vi "Autonomous Independent.vi"() -> ()   [LabVIEW 2016]
doc: "This VI is called when autonomous begins, and will automatically be terminated when autonomous ends. You can carry out timed or sensor driven robot movement independently without needing to return to the caller."
uses:
  <vilib>/Rock Robotics/WPI/Utilities/WPI_GetSetVariantRefNum.vi
  <vilib>/Rock Robotics/Network Tables/NT Read String.vi
  Robot Global Data.vi
  <vilib>/addons/control/pid/pid.llb/PID (DBL).vi
  <vilib>/Rock Robotics/Network Tables/NT Write Numeric Array.vi
  <vilib>/addons/control/pid/NI_PID_pid.lvlib
panel:
  in  "Type":bool
  in  "Range V":cluster{"output high":dbl, "output low":dbl}={"output high"=100.0, "output low"=-100.0} {"output low" format="%.2f"; "output high" format="%.2f"}
  in  "PID gains V":T1={"proportional gain (Kc)"=1.0, "integral time (Ti, min)"=0.01, "derivative time (Td, min)"=0.0} {"derivative time (Td, min)" format="%.3f"; "integral time (Ti, min)" format="%.3f"; "proportional gain (Kc)" format="%.3f"}
  in  "Range P":cluster{"output high":dbl, "output low":dbl}={"output high"=100.0, "output low"=-100.0} {"output low" format="%.2f"; "output high" format="%.2f"}
  in  "PID gains P":T1={"proportional gain (Kc)"=1.0, "integral time (Ti, min)"=0.01, "derivative time (Td, min)"=0.0} {"derivative time (Td, min)" format="%.3f"; "integral time (Ti, min)" format="%.3f"; "proportional gain (Kc)" format="%.3f"}
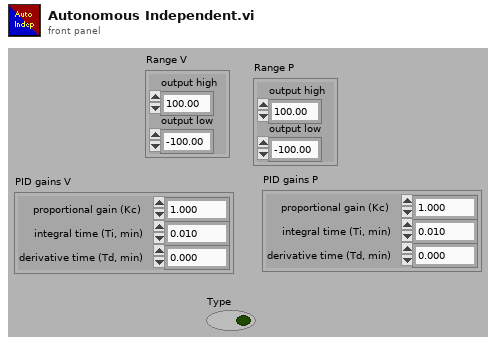
[diagram p1: front panel]
types:
  T1 = cluster{"proportional gain (Kc)":dbl, "integral time (Ti, min)":dbl, "derivative time (Td, min)":dbl}
  T2 = typedef "WPI_JoystickDevRef.ctl" = cluster{"Device":T3}
  T3 = typedef "WPI_JoystickDeviceEnum.ctl" = enum16{"USB 0", "USB 1", "USB 2", "USB 3", "USB 4", "USB 5"}
  T4 = typedef "WPI_EncoderDevRef.ctl" = cluster{"DevStatus":errorcluster, "EncoderIndex":T5, "CounterIndex":T6, "DistancePerCount":dbl, "Decoding Type":T7}
  T5 = typedef "FPGA_EncoderIdx.ctl" = enum8{"Enc 0", "Enc 1", "Enc 2", "Enc 3", "Enc 4", "Enc 5", "Enc 6", "Enc 7", "Invalid"}
  T6 = typedef "FPGA_CounterCtrSystemIndex.ctl" = enum8{"Ctr 0", "Ctr 1", "Ctr 2", "Ctr 3", "Ctr 4", "Ctr 5", "Ctr 6", "Ctr 7", "Invalid"}
  T7 = typedef "WPI_EncoderType.ctl" = enum16{"1x", "2x", "4x"}
  T8 = typedef "WPI_RobotDriveDevRef.ctl" = cluster{"DevStatus":errorcluster, "Motors[]":T9[], "Square Inputs":bool, "Max Output":dbl}
  T9 = typedef "WPI_MotorControlDeviceRef.ctl" = cluster{"DeviceStatus":errorcluster, "Type":T10, "PWM":cluster{"PWM Channel":T11, "DeadBand":T12}, "CAN":cluster{"Device Number":u8, "SetOutput VI Ref":variant, "GetOutput VI Ref":variant, "Enable VI Ref":variant, "Disable VI Ref":variant, "Data":variant}, "Invert":bool}
  T10 = typedef "WPI_MotorControlType.ctl" = enum16{"PWM", "CAN"}
  T11 = typedef "FPGA_DIOPWMChannel.ctl" = enum8{"PWM 0", "PWM 1", "PWM 2", "PWM 3", "PWM 4", "PWM 5", "PWM 6", "PWM 7", "PWM 8", "PWM 9", "PWM MXP 0", "PWM MXP 1", "PWM MXP 2", "PWM MXP 3", "PWM MXP 4", "PWM MXP 5", "PWM MXP 6", "PWM MXP 7", "PWM MXP 8", "PWM MXP 9", "Invalid"}
  T12 = typedef "WPI_PWMDeadband.ctl" = cluster{"Name":string, "maxPositivePwm":i32, "minPositivePwm":i32, "centerPwm":i32, "maxNegativePwm":i32, "minNegativePwm":i32, "angularRange":u16}
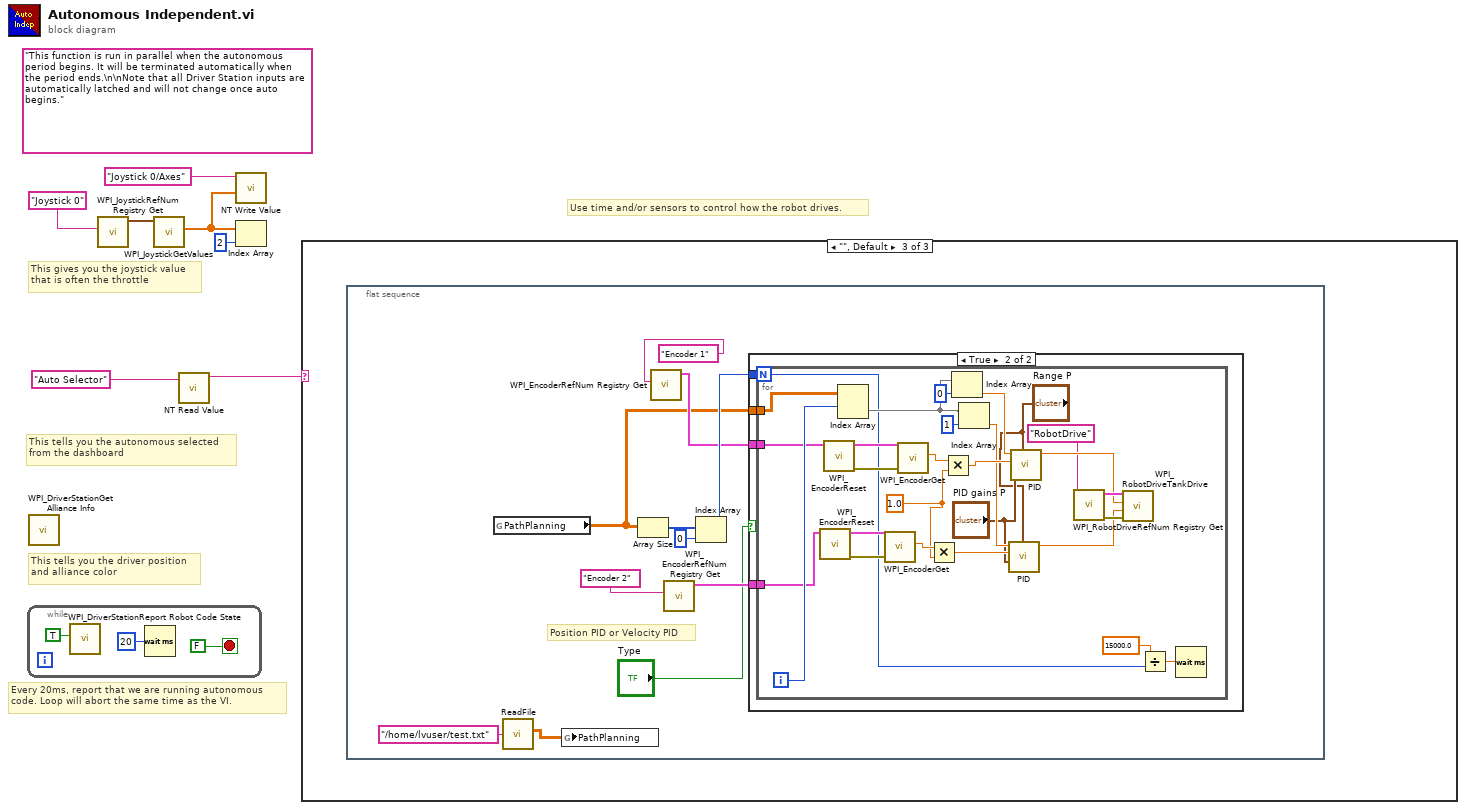
[diagram p0: block diagram]
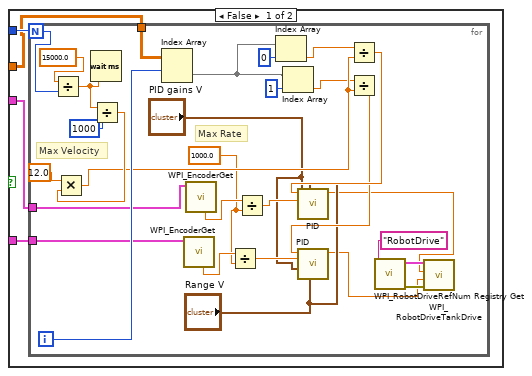
[diagram p4: hidden frame]
diagram:
  (unwired) "This function is run in parallel when the autonomous period begins. It will be terminated automatically when the period ends.\n\nNote that all Driver Station inputs are automatically latched and will not change once auto begins."
  # "This tells you the autonomous selected\nfrom the dashboard"
  # "Every 20ms, report that we are running autonomous\ncode. Loop will abort the same time as the VI."
  # "This gives you the joystick value\nthat is often the throttle"
  # "Use time and/or sensors to control how the robot drives."
  # "This tells you the driver position\nand alliance color"
  n1 = while {
    stop <- FALSE stop-if-true
    n2 = call <vilib>:"WPI_DriverStationReport Robot Code State.vi"("Autonomous"=TRUE) -> ()  [unwired: 10 in, 1 out]
    n3 = Wait (ms)(milliseconds to wait=u32 20) -> ()  [unwired: 1 out]
  }
  n4 = call <vilib>:"WPI_DriverStationGet Alliance Info.vi"() -> ()  [unwired: 12 out]
  n5 = call <vilib>:"WPI_JoystickRefNum Registry Get.vi"("refnum name"="Joystick 0") -> ("JoystickDevRef"=w6:T2)  [unwired: 1 in, 9 out]
  n6 = call <vilib>:"WPI_JoystickGetValues.vi"("JoystickDevRef"=w6) -> ("Axes"=w2:dbl[])  [unwired: 6 in, 4 out]
  n7 = call-poly <vilib>:"NT Read Value.vi"("Name"="Auto Selector") -> ("String"=w3:string)  [unwired: 9 in, 1 out]
  n8 = call-poly <vilib>:"NT Write Value.vi"("Numeric Array"=w2, "Name"="Joystick 0/Axes") -> ()  [unwired: 9 in, 1 out]
  n9 = Index Array(array=w2, index=2) -> ()  [unwired: 1 out]
  n10 = case shown="\"\", Default" w3 {
    frame "Alternative 1" {
    }
    frame "Alternative 2" {
    }
    frame "", Default {
      n11 = flat-sequence {
        frame #0 {
          # "Position PID or Velocity PID"
          n12 = global read "Robot Global Data.vi" "PathPlanning"() -> (w13:dbl[][])
          n13 = call "ReadFile.vi"("Location"="/home/lvuser/test.txt") -> ("Array - Numeric"=w11:dbl[][])  [unwired: 10 in]
          n14 = global write "Robot Global Data.vi" "PathPlanning"(w11) -> ()
          n15 = Array Size(array=w13) -> (size(s)=w21:i32[])
          n16 = call <vilib>:"WPI_EncoderRefNum Registry Get.vi"("refnum name"="Encoder 1") -> ("EncoderDevRef"=w17:T4)  [unwired: 9 in, 1 out]
          n17 = call <vilib>:"WPI_EncoderRefNum Registry Get.vi"("refnum name"="Encoder 2") -> ("EncoderDevRef"=w15:T4)  [unwired: 9 in, 1 out]
          n18 = Index Array(array=w21, index=0) -> (element=w19:i32)
          n19 = case shown="True" "Type" {
            tunnel: w13 -> [w24 w59]
            tunnel: w19 -> [w25 w58]
            tunnel: w17 -> [w23 w57]
            tunnel: w15 -> [w22 w56]
            frame False {
              n20 = for {
                N: w25 -> [w54]
                tunnel: w24 -> [w51]
                tunnel: w23 -> [w38]
                tunnel: w22 -> [w37]
                i -> [w50]
                w39 = 1000.0
                # "Max Rate"
                # "Max Velocity"
                n21 = Divide(x=15000.0, y=w54) -> (x/y=w48:dbl)
                n22 = Wait (ms)(milliseconds to wait=w48) -> ()  [unwired: 1 out]
                n23 = Divide(x=w48, y=1000) -> (x/y=w46:dbl)
                n24 = Multiply(x=12.0, y=w46) -> (x*y=w45:dbl)
                n25 = Index Array(array=w51, index (row)=w50) -> (element=w44:dbl[])  [unwired: 1 in]
                n26 = call <vilib>:"WPI_EncoderGet.vi"("EncoderDevRef"=w37) -> ("Rate"=w40:dbl)  [unwired: 5 in, 5 out]
                n27 = call <vilib>:"WPI_EncoderGet.vi"("EncoderDevRef"=w38) -> ("Rate"=w41:dbl)  [unwired: 5 in, 5 out]
                n28 = Divide(x=w40, y=w39) -> (x/y=w35:dbl)
                n29 = Divide(x=w41, y=w39) -> (x/y=w36:dbl)
                n30 = Index Array(array=w44, index=0) -> (element=w43:dbl)
                n31 = Index Array(array=w44, index=1) -> (element=w42:dbl)
                n32 = Divide(x=w43, y=w45) -> (x/y=w34:dbl)
                n33 = call-poly <vilib>:"PID.vi"("output range"="Range V", "PID gains"="PID gains V", "process variable"=w36, "setpoint"=w34) -> ("output"=w27:dbl)  [unwired: 6 in, 1 out]
                n34 = Divide(x=w42, y=w45) -> (x/y=w33:dbl)
                n35 = call-poly <vilib>:"PID.vi"("output range"="Range V", "PID gains"="PID gains V", "process variable"=w35, "setpoint"=w33) -> ("output"=w26:dbl)  [unwired: 6 in, 1 out]
                n36 = call <vilib>:"WPI_RobotDriveRefNum Registry Get.vi"("refnum name"="RobotDrive") -> ("error out"=w30:errorcluster, "RobotDriveDevRef"=w29:T8)  [unwired: 9 in]
                n37 = call <vilib>:"WPI_RobotDriveTankDrive.vi"("error in (no error)"=w30, "Right axis value"=w26, "Left axis value"=w27, "RobotDriveDevRef"=w29) -> ()  [unwired: 5 in, 3 out]
              }
            }
            frame True {
              n38 = for {
                N: w58 -> [w63]
                tunnel: w59 -> [w78]
                tunnel: w57 -> [w61]
                tunnel: w56 -> [w60]
                i -> [w77]
                w85 = 1.0
                n39 = call <vilib>:"WPI_EncoderReset.vi"("EncoderDevRef"=w60) -> ("error out"=w83:errorcluster, "EncoderDevRef"=w84:T4)  [unwired: 9 in]
                n40 = call <vilib>:"WPI_EncoderReset.vi"("EncoderDevRef"=w61) -> ("error out"=w81:errorcluster, "EncoderDevRef"=w82:T4)  [unwired: 9 in]
                n41 = Index Array(array=w78, index (row)=w77) -> (element=w74:dbl[])  [unwired: 1 in]
                n42 = call <vilib>:"WPI_EncoderGet.vi"("error in (no error)"=w83, "EncoderDevRef"=w84) -> ("Distance"=w86:dbl)  [unwired: 4 in, 5 out]
                n43 = call <vilib>:"WPI_EncoderGet.vi"("error in (no error)"=w81, "EncoderDevRef"=w82) -> ("Distance"=w87:dbl)  [unwired: 4 in, 5 out]
                n44 = Multiply(x=w86, y=w85) -> (x*y=w80:dbl)
                n45 = Multiply(x=w87, y=w85) -> (x*y=w79:dbl)
                n46 = Index Array(array=w74, index=0) -> (element=w73:dbl)
                n47 = Index Array(array=w74, index=1) -> (element=w72:dbl)
                n48 = call-poly <vilib>:"PID.vi"("output range"="Range P", "PID gains"="PID gains P", "process variable"=w80, "setpoint"=w72) -> ("output"=w67:dbl)  [unwired: 6 in, 1 out]
                n49 = call-poly <vilib>:"PID.vi"("output range"="Range P", "PID gains"="PID gains P", "process variable"=w79, "setpoint"=w73) -> ("output"=w68:dbl)  [unwired: 6 in, 1 out]
                n50 = call <vilib>:"WPI_RobotDriveRefNum Registry Get.vi"("refnum name"="RobotDrive") -> ("error out"=w70:errorcluster, "RobotDriveDevRef"=w69:T8)  [unwired: 9 in]
                n51 = call <vilib>:"WPI_RobotDriveTankDrive.vi"("error in (no error)"=w70, "Right axis value"=w67, "Left axis value"=w68, "RobotDriveDevRef"=w69) -> ()  [unwired: 5 in, 3 out]
                n52 = Divide(x=15000.0, y=w63) -> (x/y=w62:dbl)
                n53 = Wait (ms)(milliseconds to wait=w62) -> ()  [unwired: 1 out]
              }
            }
          }
        }
      }
    }
  }
